vi "Rigid Transform to Pose2d.vi"(11 "A x B":T1) -> (3 "Relative Pose":T2)   [LabVIEW 2019]
uses:
  Typedef/Pose2d.ctl
  Typedef/Translation2d.ctl
  Typedef/Rotation2d.ctl
  <vilib>/Analysis/Matrix/Datatypes/RealMatrix.ctl
  <vilib>/Analysis/Matrix/NI_Matrix.lvlib
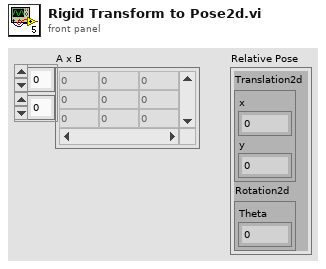
[diagram p1: front panel]
types:
  T1 = typedef "NI_Matrix.lvlib/RealMatrix.ctl" = dbl[][]
  T2 = typedef "Pose2d.ctl" = cluster{"Translation2d":T3, "Rotation2d":T4}
  T3 = typedef "Translation2d.ctl" = cluster{"x":dbl, "y":dbl}
  T4 = typedef "Rotation2d.ctl" = cluster{"Theta":dbl}
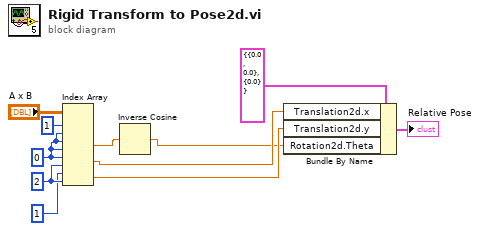
[diagram p0: block diagram]
diagram:
  w7 = 2 ("index (col)")
  w3 = 0 ("index (row)")
  n1 = Index Array(array="A x B", index (row) #1=1 ("index (row)"), index (col) #1=w3, index (row) #2=w3, index (col) #2=w3, index (row) #3=w3, index (col) #3=w7, index (row) #4=1 ("index (row)"), index (col) #4=w7) -> (element #2=w2:dbl, element #3=w10:dbl, element #4=w11:dbl)  [unwired: 1 out]
  n2 = Inverse Cosine(1:w2) -> (0:w1:dbl)
  n3 = Bundle By Name(cluster=T2 {"Translation2d"={"x"=0.0, "y"=0.0}, "Rotation2d"={"Theta"=0.0}} ("Relative Pose"), "Translation2d.x"=w10, "Translation2d.y"=w11, "Rotation2d.Theta"=w1) -> (→"Relative Pose":T2)
